vi "Solve2.vi"(8 "Error In":errorcluster, 11 "object in":refnum<class "2024_16.lvclass">) -> (0 "Error Out":errorcluster, 2 "Result":u64, 3 "object out":refnum<class "2024_16.lvclass">)   [LabVIEW 2023, in "2024_16.lvclass"]
uses:
  2024_16.lvclass
  Tile.ctl
  2024_16.lvclass/2024_16.ctl
  Common/AOC_Direction.ctl
  Common/AOC_XY(I32).ctl
panel:
  out "Array":u32[][](array[colorbox])
  out "size(s)":i32
  out "map":T1[][](array[typedef])
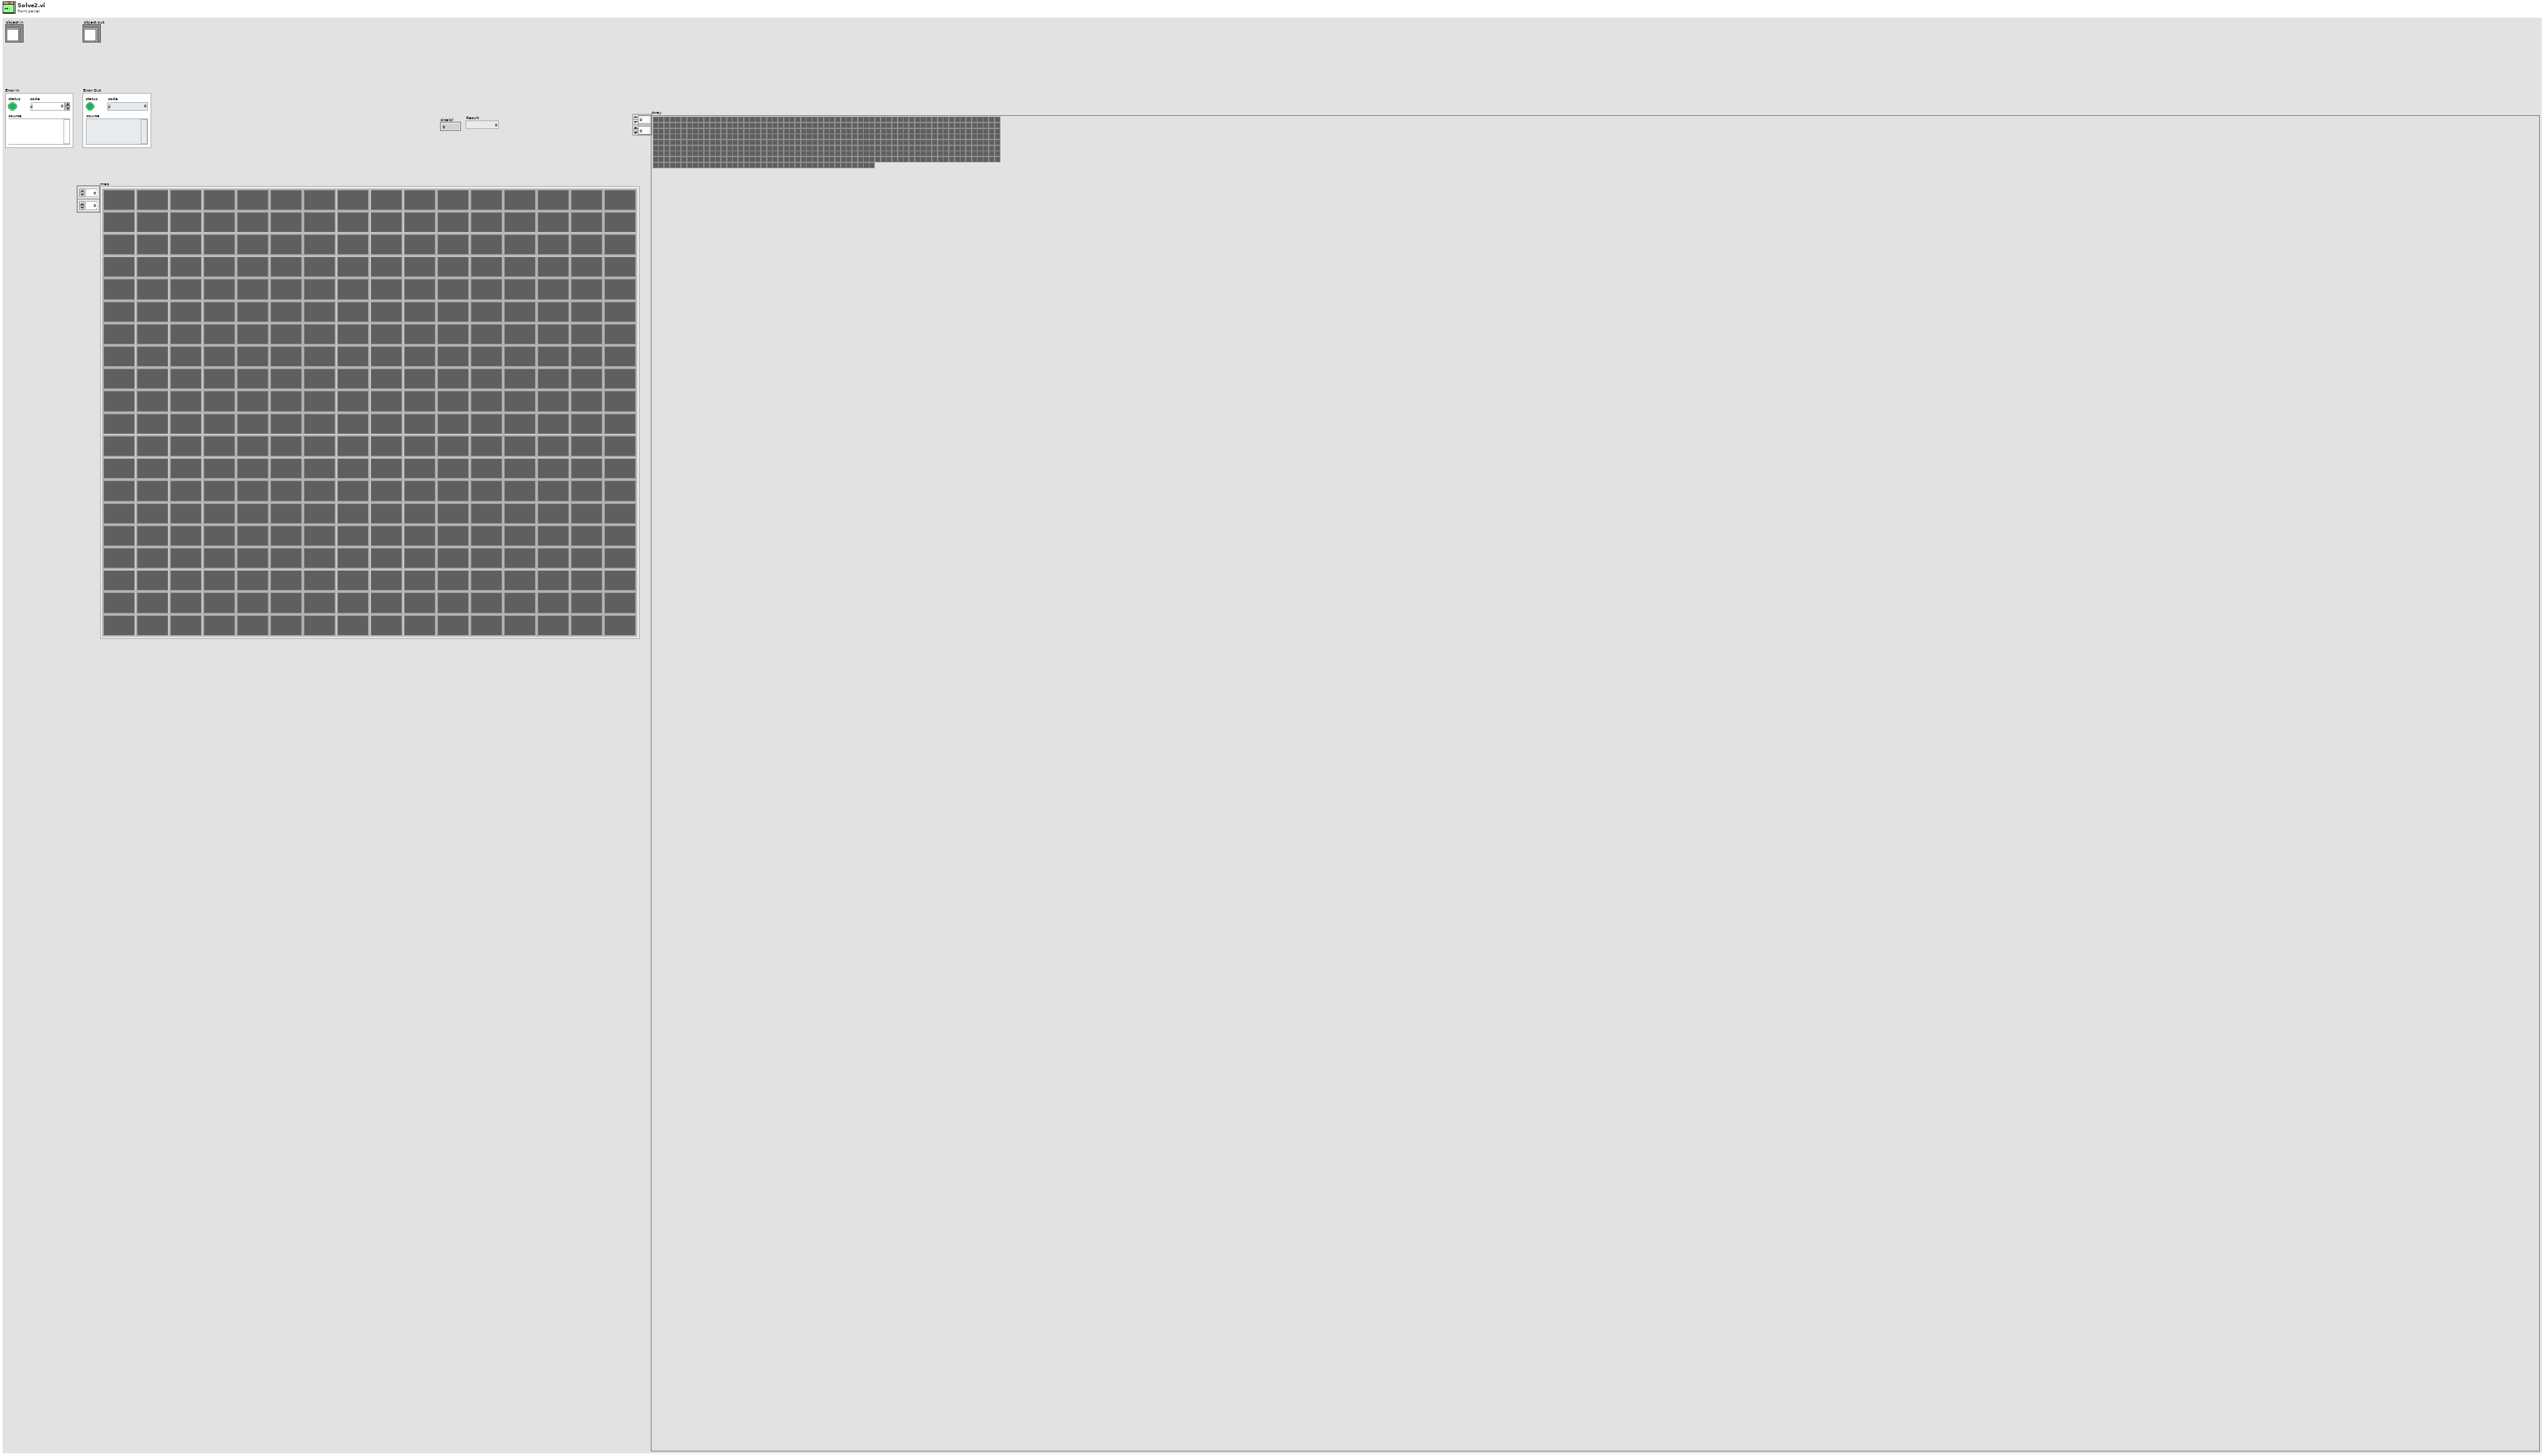
[diagram p1: front panel]
types:
  T1 = typedef "2024_16.lvclass/Tile.ctl" = cluster{"Up":i32, "Right":i32, "Down":i32, "Left":i32, "BGColor":u32}
  T2 = typedef "AOC_Direction.ctl" = enum16{"Up", "Right", "Down", "Left"}
  T3 = typedef "AOC_XY(I32).ctl" = cluster{"X":i32, "Y":i32}
  T4 = map{T3, cluster{"Up":u64, "Right":u64, "Down":u64, "Left":u64}}
  T5 = cluster{"Up":u64, "Right":u64, "Down":u64, "Left":u64}
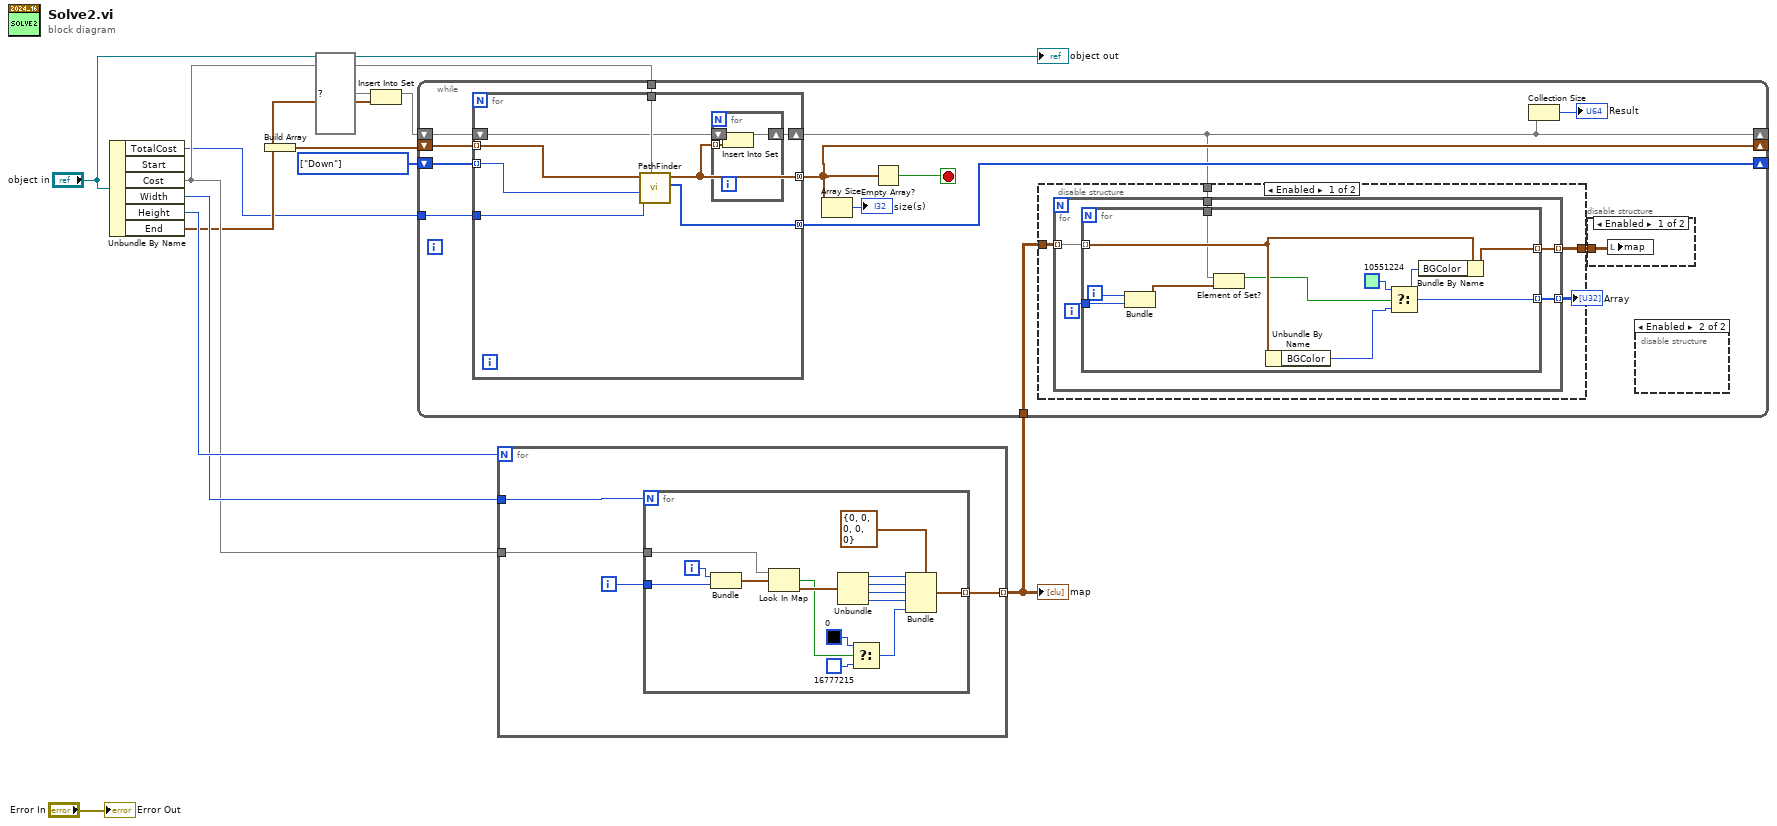
[diagram p0: block diagram]
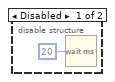
[diagram p4: hidden frame]
diagram:
  w2 = T2[] [enum."Down"] items=["Up", "Right", "Down", "Left"] ("Directions")
  n1 = Unbundle By Name("object in") -> ("TotalCost"=w1:u64, "Cost"=w8:T4, "Width"=w9:i32, "Height"=w10:i32, "End"=w3:T3)  [unwired: 1 out]
  n2 = Build Array(w3) -> (w6:T3[])
  n3 = Insert Into Set(10:w3, 11:set{T3} {} ("set in")) -> (3:w4:set{T3})  [unwired: 1 out]
  n4 = for {
    N: w10 -> [_]
    tunnel: w9 -> [w16]
    tunnel: w8 -> [w14]
    tunnel: [w13] -> w7 mode=indexing
    i -> [w15]
    n5 = for {
      N: w16 -> [_]
      tunnel: w15 -> [w30]
      tunnel: w14 -> [w29]
      tunnel: [w17] -> w13 mode=indexing
      i -> [w31]
      n6 = Bundle(w31, w30) -> (w28:cluster{i32, i32})  [unwired: 1 in]
      n7 = Look In Map(map=w29, key=w28) -> (key not found?=w21:bool, value=w27:T5)  [unwired: 1 in]
      n8 = Unbundle(w27) -> ("Up"=w25:u64, "Right"=w24:u64, "Down"=w23:u64, "Left"=w22:u64)
      n9 = Select(t=u32 0 ("BGColor"), s=w21, f=u32 16777215 ("BGColor")) -> (s? t:f=w18:u32)
      n10 = Bundle(cluster=T1 {"Up"=0, "Right"=0, "Down"=0, "Left"=0, "BGColor"=0} ("Cluster"), "Up"=w25, "Right"=w24, "Down"=w23, "Left"=w22, "BGColor"=w18) -> (w17:T1)
    }
  }
  "map" <- w7
  n11 = while {
    tunnel: w8 -> [w44]
    tunnel: w1 -> [w43]
    shift-right: [w35] -> _
    shift-left: w6 -> [w42]
    tunnel: w7 -> [w41]
    shift-right: [w32] -> _
    shift-left: w4 -> [w39]
    shift-right: [w37] -> _
    shift-left: w2 -> [w36]
    stop <- w38 stop-if-true
    n12 = for {
      tunnel: w44 -> [w73]
      tunnel: w43 -> [w66]
      tunnel: w42 -> [w72] mode=indexing
      tunnel: [w71] -> w35 mode=concatenating
      shift-right: [w69] -> w32
      shift-left: w39 -> [w70]
      tunnel: [w68] -> w37 mode=concatenating
      tunnel: w36 -> [w67] mode=indexing
      n13 = call "PathFinder.vi"("Cost"=w73, "TotalCost"=w66, "Direction"=w67, "AnalysePosition"=w72) -> ("Directions"=w68:T2[], "Positions"=w71:T3[])  [unwired: 6 in]
      n14 = for {
        tunnel: w71 -> [w76] mode=indexing
        shift-right: [w74] -> w69
        shift-left: w70 -> [w75]
        n15 = Insert Into Set(10:w76, 11:w75) -> (3:w74:set{T3})  [unwired: 1 out]
      }
    }
    n16 = Array Size(array=w35) -> (size(s)=→"size(s)":i32)
    n17 = Empty Array?(array=w35) -> (empty?=w38:bool)
    n18 = disable-structure shown="Enabled" {
      disable-tunnel: w41 -> [w48 _]
      disable-tunnel: [w47 _] -> w40
      disable-tunnel: w32 -> [w46 _]
      frame Enabled {
        n19 = for {
          tunnel: w48 -> [w53] mode=indexing
          tunnel: [w51] -> w47 mode=indexing
          tunnel: w46 -> [w50]
          tunnel: [w49] -> w45 mode=indexing
          i -> [w52]
          n20 = for {
            tunnel: w53 -> [w59] mode=indexing
            tunnel: w52 -> [w62]
            tunnel: [w61] -> w51 mode=indexing
            tunnel: w50 -> [w57]
            tunnel: [w54] -> w49 mode=indexing
            i -> [w63]
            n21 = Bundle(w63, w62) -> (w56:cluster{i32, i32})  [unwired: 1 in]
            n22 = Element of Set?(10:w56, 11:w57) -> (3:w55:bool)
            n23 = Unbundle By Name(w59) -> ("BGColor"=w58:u32)
            n24 = Select(t=u32 10551224 ("BGColor"), s=w55, f=w58) -> (s? t:f=w54:u32)
            n25 = Bundle By Name(cluster=w59, "BGColor"=w54) -> (w61:T1)
          }
        }
        "Array" <- w45
      }
      frame Disabled {
      }
    }
    n26 = Collection Size(1:w32) -> (0:→"Result":i32)
    n27 = disable-structure shown="Enabled" {
      disable-tunnel: w40 -> [w64 _]
      frame Enabled {
        n28 = local write "map"(w64) -> ()
      }
      frame Disabled {
      }
    }
    n29 = disable-structure shown="Enabled" {
      frame Disabled {
        n30 = Wait (ms)(milliseconds to wait=u32 20) -> ()  [unwired: 1 out]
      }
      frame Enabled {
      }
    }
  }
  "Error Out" <- "Error In"
  "object out" <- "object in"
